vi "virtual_temp.vi"() -> ()   [LabVIEW 2019]
panel:
  out "Waveform Graph":dynamicdata(graph)
  out "Array 2":dbl[](array[knob]) scale=0.0..50.0
  out "Array":dbl[](array[slide]) scale=0.0..100.0
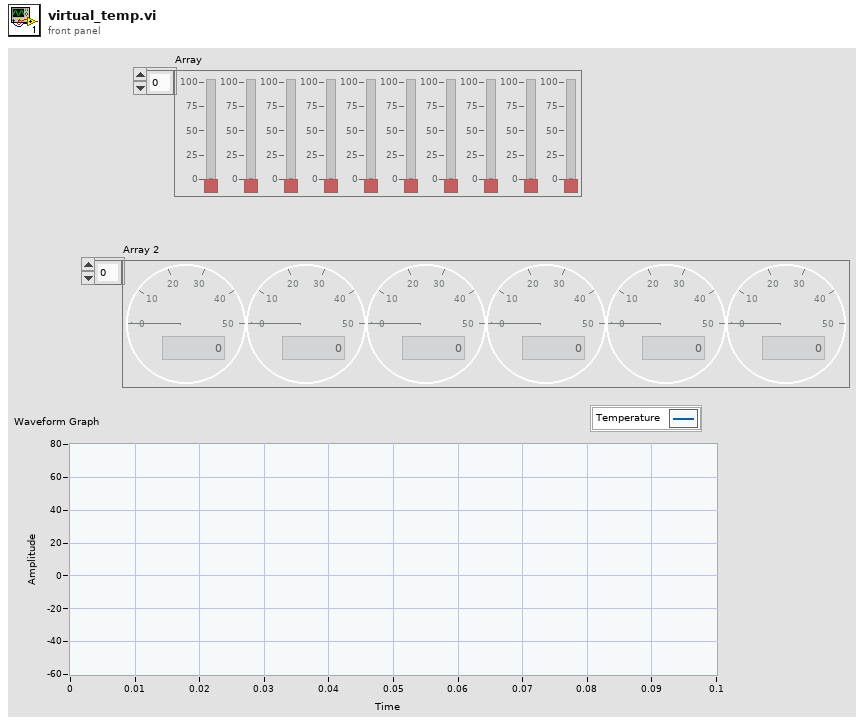
[diagram p1: front panel]
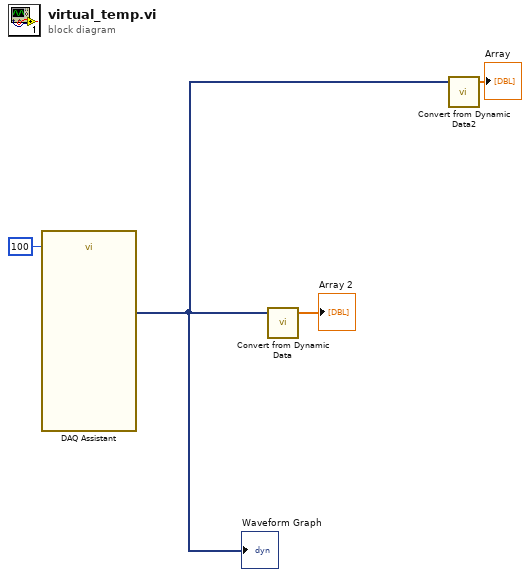
[diagram p0: block diagram]
diagram:
  n1 = call "DAQ Assistant"("number of samples"=100) -> ("data"=w2:dynamicdata)  [unwired: 16 in, 2 out]
  "Waveform Graph" <- w2
  n2 = call "Convert from Dynamic Data"("Dynamic Data Type"=w2) -> ("Array"=→"Array 2":dbl[])  [unwired: 3 in]
  n3 = call "Convert from Dynamic Data2"("Dynamic Data Type"=w2) -> ("Array"=→"Array":dbl[])  [unwired: 3 in]
